vi "TempForLoopShift.vi"() -> ()   [LabVIEW 2015]
uses:
  <vilib>/measure/NI_MABase.lvlib
panel:
  out "Overall Avg Temp (Deg F)":dbl(graph)
  out "Overall Avg Temp (Deg F)":dbl
  out "Two Point Avg Temprature (Deg F)":dbl(graph)
  out "Two Point Avg Temp (Deg F)":dbl
  out "Current Temp (Deg F)":dbl
  out "Current Elapsed \nTime (sec)":dbl
  out "Temperature (Deg F)":dbl(graph)
  in  "Input Temp Scale":bool
  in  "?":dbl
  in  "?":dbl
  # "Input desired duration of measurements in seconds"
  # "Input desired Time Measurement Intervals in seconds"
  # "Indicate Temperature Scale of Measuring Device"
  # "Deg C\nDeg F"
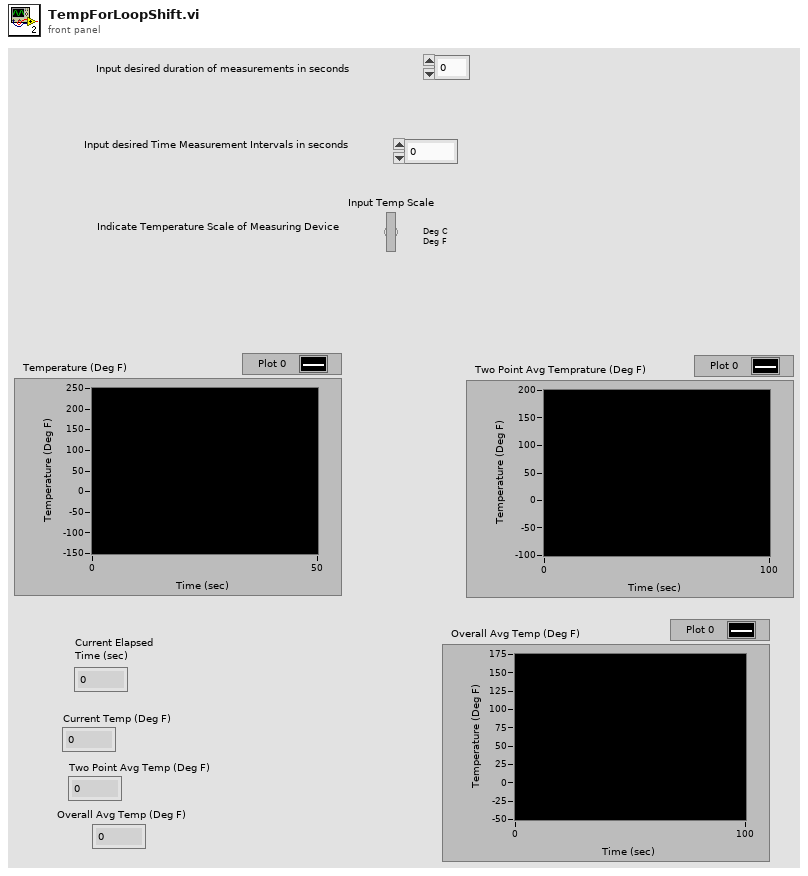
[diagram p1: front panel]
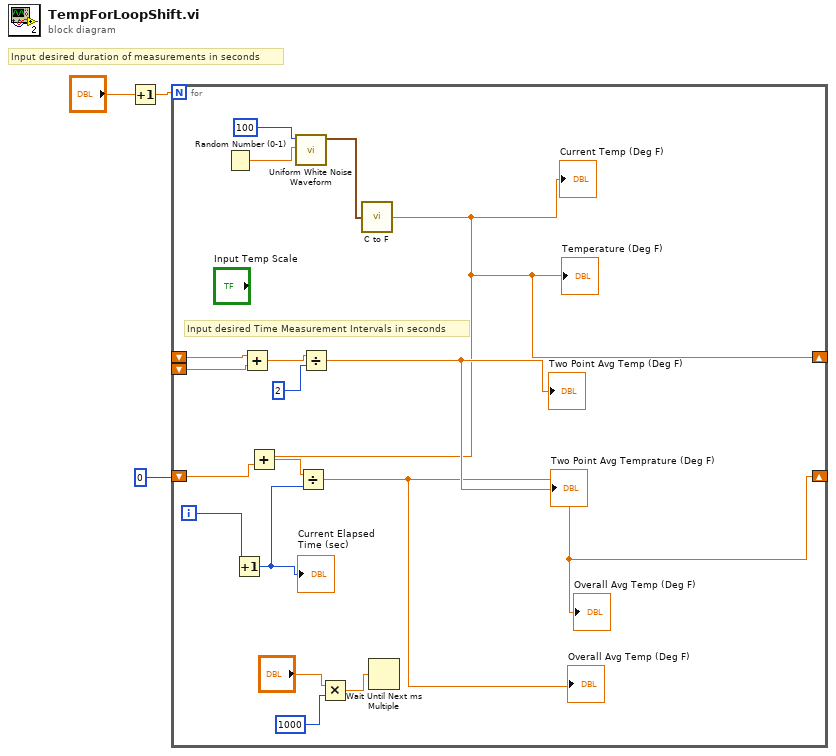
[diagram p0: block diagram]
diagram:
  # "Input desired duration of measurements in seconds"
  n1 = Increment(x="?") -> (x+1=w2:dbl)
  n2 = for {
    N: w2 -> [_]
    shift-right: [w8] -> _
    shift-left: _ -> [w13]
    shift-left: _ -> [w12]
    shift-right: [w4] -> _
    shift-left: 0 -> [w7]
    i -> [w14]
    # "Input desired Time Measurement Intervals in seconds"
    n3 = Random Number (0-1)() -> (number: 0 to 1=w20:dbl)
    n4 = Increment(x=w14) -> (x+1=w5:i32)
    "Current Elapsed \nTime (sec)" <- w5
    n5 = Add(x=w13, y=w12) -> (x+y=w11:dbl)
    n6 = call <vilib>:"Uniform White Noise Waveform.vi"("seed"=w20, "amplitude"=100) -> ("signal out"=w18:waveform(dbl))  [unwired: 8 in, 1 out]
    n7 = Divide(x=w11, y=2) -> (x/y=→"Two Point Avg Temp (Deg F)" →"Two Point Avg Temprature (Deg F)":dbl)
    n8 = Multiply(x="?", y=1000) -> (x*y=w15:dbl)
    n9 = call "C to F.vi"("DEG C"=w18) -> ("Deg F"=w8:dbl)
    "Current Temp (Deg F)" <- w8
    "Temperature (Deg F)" <- w8
    n10 = Add(x=w8, y=w7) -> (x+y=w6:dbl)
    n11 = Divide(x=w6, y=w5) -> (x/y=w4:dbl)
    "Overall Avg Temp (Deg F)" <- w4
    "Overall Avg Temp (Deg F)" <- w4
    n12 = Wait Until Next ms Multiple(millisecond multiple=w15) -> ()  [unwired: 1 out]
  }
